vi "load_bin_trace.vi"(4 "Last offset":i64=-1, 6 "Start offset":i64=12, 8 "error in":errorcluster, 10 "File path":path) -> (0 "error out":errorcluster, 2 "Output data":sgl[][][](array[numeric]))   [LabVIEW 2013]
panel:
  # "Read in trace data, returning it directly, and also storing it as though it was a new trace for select_waveforms.vi, etc."
  # "Byte offsets in data file of the starts of the first and last records to read.  Defaults are to start at the first record and read the remainder of file."
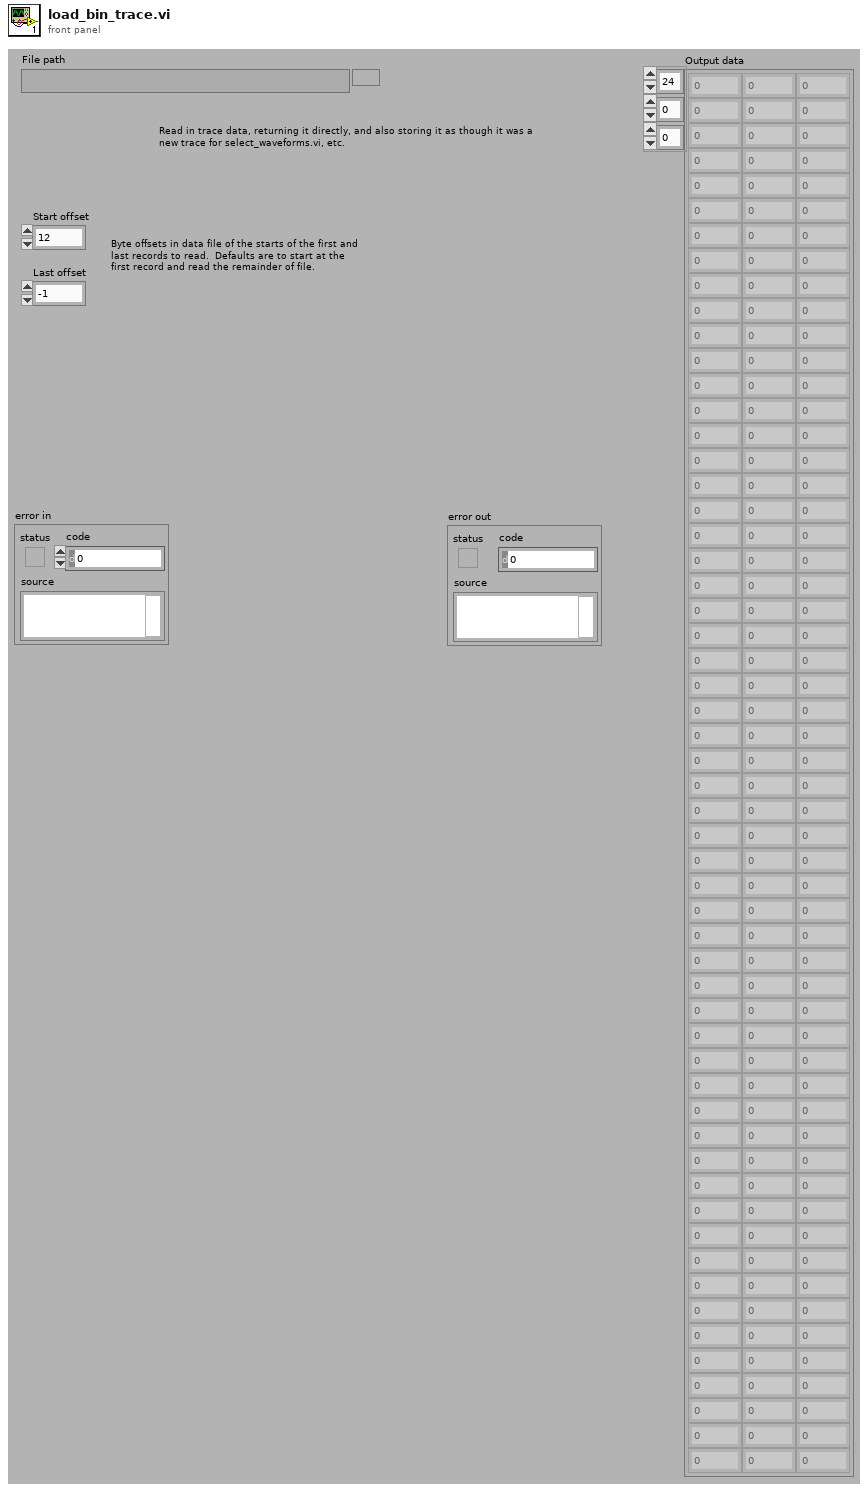
[diagram p1: front panel]
types:
  T1 = enum16{"big-endian, network order", "native, host order", "little-endian"}
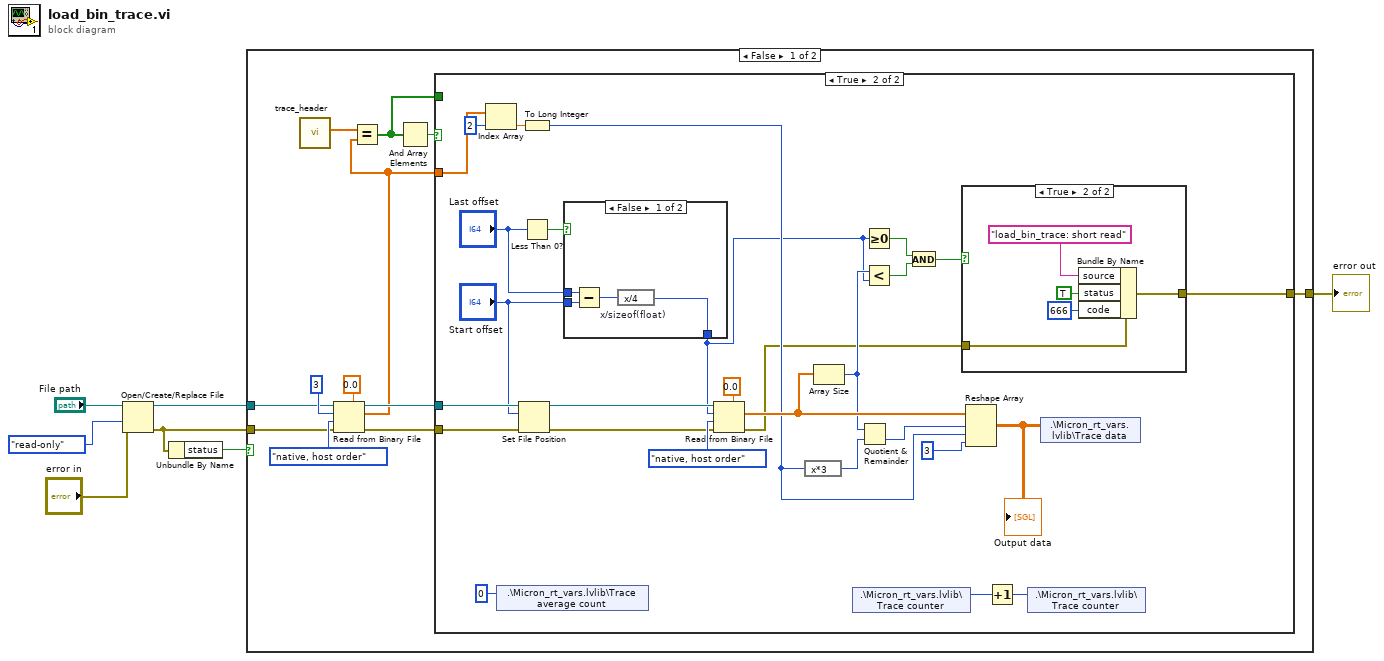
[diagram p0: block diagram]
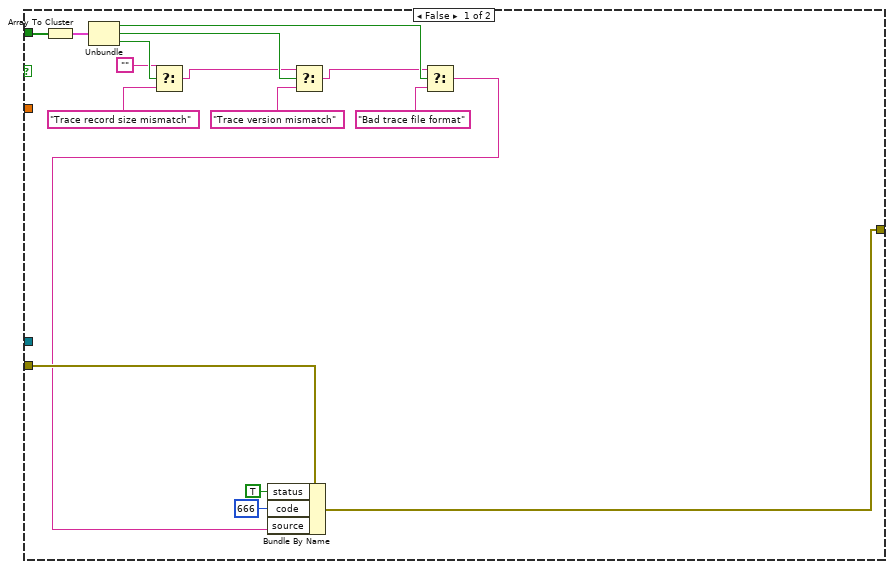
[diagram p2: hidden frame]
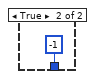
[diagram p4: hidden frame]
diagram:
  n1 = Open/Create/Replace File(file path (use dialog)="File path", error in="error in", access (0:read/write)=enum16{"read/write", "read-only", "write-only"}."read-only") -> (refnum out=w4:refnum<file>, error out=w3:errorcluster)  [unwired: 3 in, 1 out]
  n2 = Unbundle By Name(w3) -> ("status"=w2:bool)
  n3 = case shown="False" w2 {
    tunnel: w4 -> [w15 _]
    tunnel: w3 -> [w14 w75]
    tunnel: [w8 w75] -> w1
    frame False {
      n4 = call "trace_header.vi"() -> ("Header"=w16:sgl[])  [unwired: 11 in]
      n5 = Read from Binary File(5:sgl 0.0, 8:w14, 9:T1."native, host order" ("byte order (0:big-endian, network order)"), 10:3 ("count (1)"), 11:w15) -> (0:w12:errorcluster, 2:w11:sgl[], 3:w13:refnum<file>)  [unwired: 1 in, 1 out]
      n6 = Equal?(x=w16, y=w11) -> (x = y?=w9:bool[])
      n7 = And Array Elements(Boolean array=w9) -> (logical AND=w10:bool)
      n8 = case shown="True" w10 {
        tunnel: w11 -> [_ w51]
        tunnel: w13 -> [_ w54]
        tunnel: w12 -> [w35 w55]
        tunnel: w9 -> [w32 _]
        tunnel: [w20 w36] -> w8
        frame False {
          n9 = Array To Cluster(array=w32) -> (cluster=w31:cluster{"[0]":bool, "[1]":bool, "[2]":bool})
          n10 = Unbundle(w31) -> ("[0]"=w29:bool, "[1]"=w27:bool, "[2]"=w25:bool)
          n11 = Select(t="", s=w25, f="Trace record size mismatch" ("source")) -> (s? t:f=w23:string)
          n12 = Select(t=w23, s=w27, f="Trace version mismatch" ("source")) -> (s? t:f=w22:string)
          n13 = Select(t=w22, s=w29, f="Bad trace file format" ("source")) -> (s? t:f=w21:string)
          n14 = Bundle By Name(cluster=w35, "status"=TRUE, "code"=666, "source"=w21) -> (w20:errorcluster)
        }
        frame True {
          n15 = Index Array(array=w51, index=2) -> (element=w62:sgl)
          n16 = shared-variable ".\\Micron_rt_vars.lvlib\\Trace average count"(u32 0 ("Trace average count")) -> ()  [unwired: 2 out]
          n17 = Set File Position(offset (in bytes) (0)="Start offset", refnum=w54, error in=w55) -> (refnum out=w46:refnum<file>, error out=w47:errorcluster)  [unwired: 1 in]
          n18 = To Long Integer(number=w62) -> (32bit integer=w43:i32)
          n19 = Less Than 0?(x="Last offset") -> (x < 0?=w48:bool)
          n20 = case shown="False" w48 {
            tunnel: "Start offset" -> [w72 _]
            tunnel: [w70 i64 -1] -> w39
            tunnel: "Last offset" -> [w71 _]
            frame False {
              n21 = Subtract(x=w71, y=w72) -> (x-y=w73:i64)
              n22 = expression code="x/4" "x/sizeof(float)"(w73) -> (w70:i64)
            }
            frame True {
            }
          }
          n23 = Read from Binary File(5:sgl 0.0, 8:w47, 9:T1."native, host order" ("byte order (0:big-endian, network order)"), 10:w39, 11:w46) -> (0:w37:errorcluster, 2:w45:sgl[])  [unwired: 1 in, 2 out]
          n24 = expression code="x*3" ("x/sizeof(float)")(w43) -> (w44:i32)
          n25 = Array Size(array=w45) -> (size(s)=w40:i32)
          n26 = shared-variable ".\\Micron_rt_vars.lvlib\\Trace counter"() -> (w59:u32)  [unwired: 2 out]
          n27 = Quotient & Remainder(x=w40, y=w44) -> (floor(x/y)=w56:i32)  [unwired: 1 out]
          n28 = Greater Or Equal To 0?(x=w39) -> (x >= 0?=w42:bool)
          n29 = Less?(x=w40, y=w39) -> (x < y?=w41:bool)
          n30 = And(x=w42, y=w41) -> (x .and. y?=w38:bool)
          n31 = case shown="True" w38 {
            tunnel: w37 -> [w64 w69]
            tunnel: [w64 w65] -> w36
            frame False {
            }
            frame True {
              n32 = Bundle By Name(cluster=w69, "source"="load_bin_trace: short read", "status"=TRUE, "code"=666) -> (w65:errorcluster)
            }
          }
          n33 = Reshape Array(w45, w56, w43, 3 ("dimension size")) -> (w60:sgl[][][])
          "Output data" <- w60
          n34 = Increment(x=w59) -> (x+1=w58:u32)
          n35 = shared-variable ".\\Micron_rt_vars.lvlib\\Trace counter"(w58) -> ()  [unwired: 2 out]
          n36 = shared-variable ".\\Micron_rt_vars.lvlib\\Trace data"(w60) -> ()  [unwired: 2 out]
        }
      }
    }
    frame True {
    }
  }
  "error out" <- w1
